vi "Get Palettes.vi"(8 "error in (no error)":errorcluster, 11 "Material Theme in":refnum<class "Material Theme.lvclass">) -> (0 "error out":errorcluster, 2 "Material-Palettes":refnum<class "Material-Palette.lvclass">[](array[class]), 3 "Material Theme out":refnum<class "Material Theme.lvclass">)   [LabVIEW 2021, in "TSC Material Theme.lvlib" / "Material Theme.lvclass"]
doc: "Get the defined scheme from the loaded theme\n\n<b>Code Developed By:</b> +\nDaniel Coons +\nTechnology Service Corporation +\nwww.tsc.com/atcs"
uses:
  Material Theme.lvclass
  Material-Palette/Material-Palette.lvclass
  Material Theme.lvclass/Material Theme.ctl
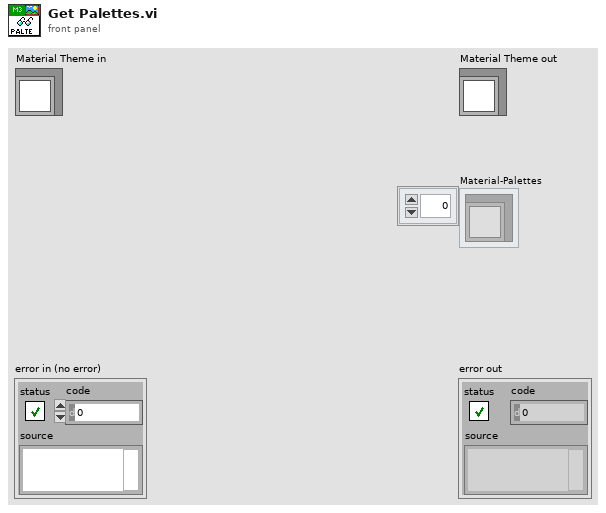
[diagram p1: front panel]
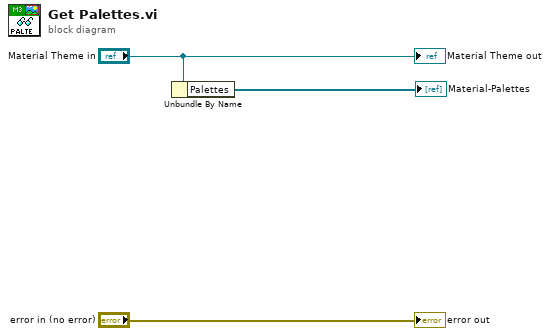
[diagram p0: block diagram]
diagram:
  n1 = Unbundle By Name("Material Theme in") -> ("Palettes"=→"Material-Palettes":refnum<class "Material-Palette.lvclass">[])
  "error out" <- "error in (no error)"
  "Material Theme out" <- "Material Theme in"
